vi "Render Unescaped Tag-Text.vi"(8 "Error In":errorcluster) -> (0 "Error Out":errorcluster)   [LabVIEW 2018, in "Tests.lvlib" / "Render.lvlib"]
uses:
  Render.lvlib
  <vilib>/addons/_JKI Toolkits/Caraya/classes/Test/Test.lvclass
  <vilib>/addons/_JKI Toolkits/Caraya/classes/Assert/Assert.lvclass
  src/Toolkit/Low-Level/Renderer/Abstract/Render to String.vi
  src/Toolkit/Low-Level/Support/Lex String.vi
  src/Toolkit/Data/Pair/Pair.lvclass
  src/Toolkit/Data/Pair/Support/From String.vi
  src/Toolkit/Low-Level/Compiler/Compiler.lvclass
  D:/Users/cfield/Code/Field R&D Services/Labstache/src/Toolkit/Data/Datum/Datum.lvclass
  src/Toolkit/Low-Level/Nodes/Root/Root.lvclass
  D:/Users/cfield/Code/Field R&D Services/Labstache/src/Toolkit/Low-Level/Nodes/NonTerminal/NonTerminal.lvclass
  D:/Users/cfield/Code/Field R&D Services/Labstache/src/Toolkit/Low-Level/Nodes/Node/Node.lvclass
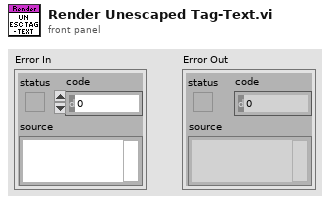
[diagram p1: front panel]
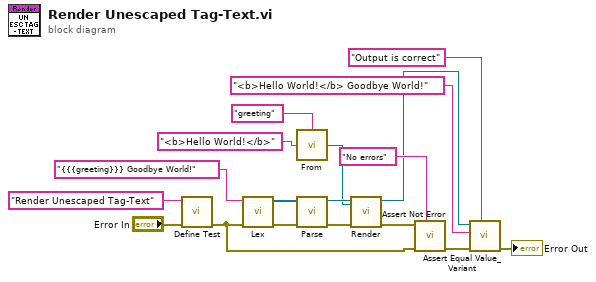
[diagram p0: block diagram]
diagram:
  n1 = call <vilib>:"Define Test.vi"("error in (no error)"="Error In", "Label (VI Title)"="Render Unescaped Tag-Text") -> ("error out"=w4:errorcluster)  [unwired: 9 in]
  n2 = call-poly "Lex.vi"("Error In"=w4, "Input"="{{{greeting}}} Goodbye World!" ("format string")) -> ("Error Out"=w7:errorcluster, "Tokens"=w8:refnum<class "Token.lvclass">[])  [unwired: 8 in]
  n3 = call-poly "From.vi"("Value"="<b>Hello World!</b>", "Key"="greeting") -> ("Pair"=w1:refnum<class "Pair.lvclass">)
  n4 = call "Parse.vi"("Error In"=w7, "Tokens"=w8) -> ("Error Out"=w9:errorcluster, "Abstract Syntax Tree"=w10:refnum<class "Root.lvclass">)  [unwired: 8 in]
  n5 = call-poly "Render.vi"(7:w1, "Error In"=w9, "Context In"=w10) -> ("Error Out"=w12:errorcluster, "Context Out"=w5:refnum<class "Compiler.lvclass">)  [unwired: 6 in, 1 out]
  n6 = call <vilib>:"Assert Not Error.vi"("Label"="No errors", "error in (no error)"=w4, "Not Error?"=w12) -> ("error out"=w15:errorcluster)  [unwired: 8 in]
  n7 = call <vilib>:"Assert Equal Value_Variant.vi"("Label"="Output is correct", "error in (no error)"=w15, "Y"="<b>Hello World!</b> Goodbye World!", "X"=w5) -> ("error out"=→"Error Out":errorcluster)  [unwired: 7 in]
